vi "Read Initialized.vi"(8 "error in (no error)":errorcluster, 11 "DigitizerBase in":refnum<class "DigitizerBase.lvclass">) -> (0 "error out":errorcluster, 2 "Initialized":bool, 3 "DigitizerBase out":refnum<class "DigitizerBase.lvclass">)   [LabVIEW 2018, in "DigitizerPlugins.lvlib" / "DigitizerBase.lvclass"]
uses:
  DigitizerBase.lvclass
  DigitizerBase.lvclass/DigitizerBase.ctl
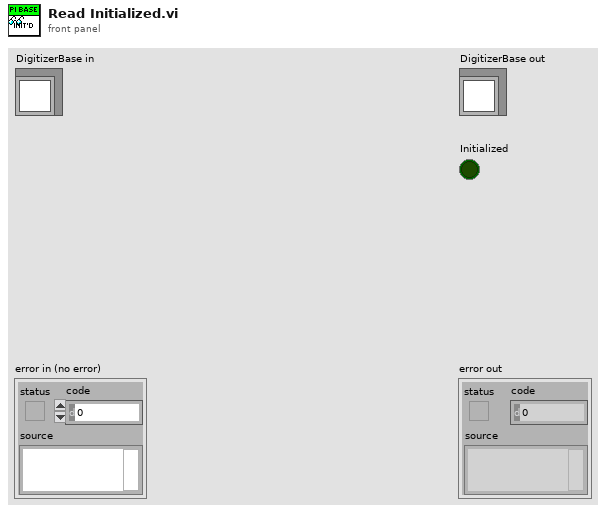
[diagram p1: front panel]
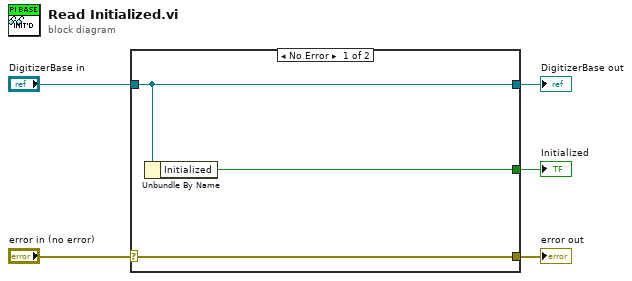
[diagram p0: block diagram]
diagram:
  n1 = case shown="No Error" "error in (no error)" {
    selector: "error in (no error)" -> [w8 w9]
    tunnel: [w8 w9] -> w4
    tunnel: [w7 w10] -> w2
    tunnel: "DigitizerBase in" -> [w7 w10]
    tunnel: [w6 _] -> w1
    frame No Error {
      n2 = Unbundle By Name(w7) -> ("Initialized"=w6:bool)
    }
    frame Error {
    }
  }
  "error out" <- w4
  "DigitizerBase out" <- w2
  "Initialized" <- w1
